vi "Read Server RPC Methods.vi"(8 "error in (no error)":errorcluster, 11 "SignalGeneratorService in":refnum<class "Greeter.lvclass">=refnum) -> (0 "error out":errorcluster, 2 "Server RPC Methods":T1, 3 "SignalGeneratorService out":refnum<class "Greeter.lvclass">)   [LabVIEW 2019, in "helloworld_server.lvlib" / "Greeter.lvclass"]
uses:
  Greeter.lvclass
  Greeter.lvclass/Greeter.ctl
  typeDefs/Server gRPC UEs.ctl
  labview source/gRPC lv Support/grpc-lvsupport/gRPCId Cluster.ctl
  labview source/gRPC lv Support/grpc-lvsupport/grpc-lvsupport.lvlib
  labview source/gRPC lv Support/grpc-lvsupport/grpcId.ctl
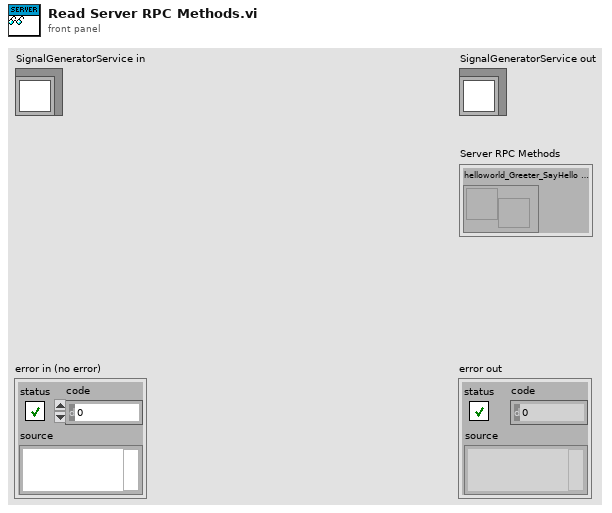
[diagram p1: front panel]
types:
  T1 = typedef "helloworld_server.lvlib/Greeter.lvclass/Server gRPC UEs.ctl" = cluster{"helloworld_Greeter_SayHello gRPC UE":refnum<user-event>}
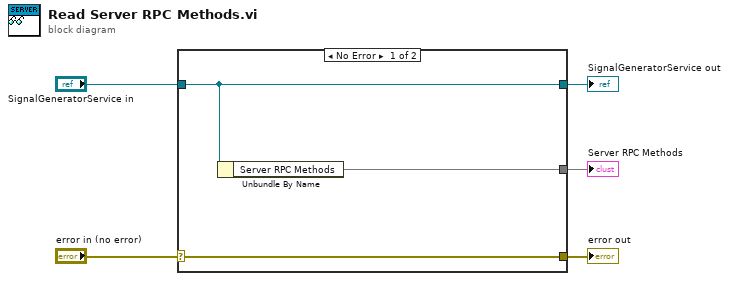
[diagram p0: block diagram]
diagram:
  n1 = case shown="No Error" "error in (no error)" {
    selector: "error in (no error)" -> [w8 w9]
    tunnel: [w8 w9] -> w4
    tunnel: [w7 w10] -> w2
    tunnel: "SignalGeneratorService in" -> [w7 w10]
    tunnel: [w6 _] -> w1
    frame No Error {
      n2 = Unbundle By Name(w7) -> ("Server RPC Methods"=w6)
    }
    frame Error {
    }
  }
  "error out" <- w4
  "SignalGeneratorService out" <- w2
  "Server RPC Methods" <- w1
